vi "svx_Oct_Crop X to scale.vi"(7 "Display State In":T1={"X Scale Width %"=50.0, "Y Scale Height %"=50.0, "X-Axis Range"={"Minimum"=0.0, "Maximum"=10.0}, "Y-Axis Range"={"Minimum"=0.0, "Maximum"=10.0}, "Z-Axis Range"={"Minimum"=0.0, "Maximum"=10.0}, "Plot Color"=0, "Frame Color"=61212, "Background Color"=16252785, "Initial AutoScale Y"=TRUE, "AutoScale X"=2, "AutoScale Y"=2, "AutoScale Z"=2, "Plot Transparency"=FALSE, "X-Axis Name"="Frequency", "Y-Axis Name"="Amplitude", "Z-Axis Name"="", "X-Axis Scaling Factor"={"Offset"=0.0, "Multiplier"=1.0}, "Y-Axis Scaling Factor"={"Offset"=0.0, "Multiplier"=1.0}, "Z-Axis Scaling Factor"={"Offset"=0.0, "Multiplier"=1.0}, "X-Scale Visible"=TRUE, "Y-Scale Visible"=TRUE, "Z-Scale Visible"=TRUE, "X-Scale Label Visible"=TRUE, "Y-Scale Label Visible"=TRUE, "Z-Scale Label Visible"=TRUE, "X-Axis Range Scaled"={"Minimum"=0.0, "Maximum"=10.0}, "Y-Axis Range Scaled"={"Minimum"=0.0, "Maximum"=10.0}, "Z-Axis Range Scaled"={"Minimum"=0.0, "Maximum"=10.0}, "Rev Z Order"=FALSE, "X-Scale Format Str"="%#.4g", "Y-Scale Format Str"="%#.4g", "Z-Scale Format Str"="%#.4g", "Decor color"=12369084, "Scale Range Change"=refnum, "out of state queue"=refnum, "property nodes"=refnum} caption="State", 9 "Cropped Info":cluster{"First Index":i32, "Length":i32}, 11 "Waveform Array In":T2={"z0"=0.0, "dz"=1.0, "Plots"=[]} {"Plots"."Y" format="%.2f"; "Plots"."X" format="%.2f"}) -> (1 "Cropped Info out":cluster{"First Index":i32, "Length":i32}, 3 "Waveform Array Out":T2={"z0"=0.0, "dz"=1.0, "Plots"=[]} {"Plots"."Y" format="%.2f"; "Plots"."X" format="%.2f"})   [LabVIEW 2017, in "SVX Octave Waterfall Graph.xctl"]
uses:
  <vilib>/addons/_XControls/Octave Waterfall Graph/SVX Octave Waterfall Graph.xctl
  <vilib>/addons/_XControls/Octave Waterfall Graph/subVIs/svx_Oct_Waterfall Data.ctl
  <vilib>/addons/_XControls/Octave Waterfall Graph/subVIs/svx_Oct_Waterfall State.ctl
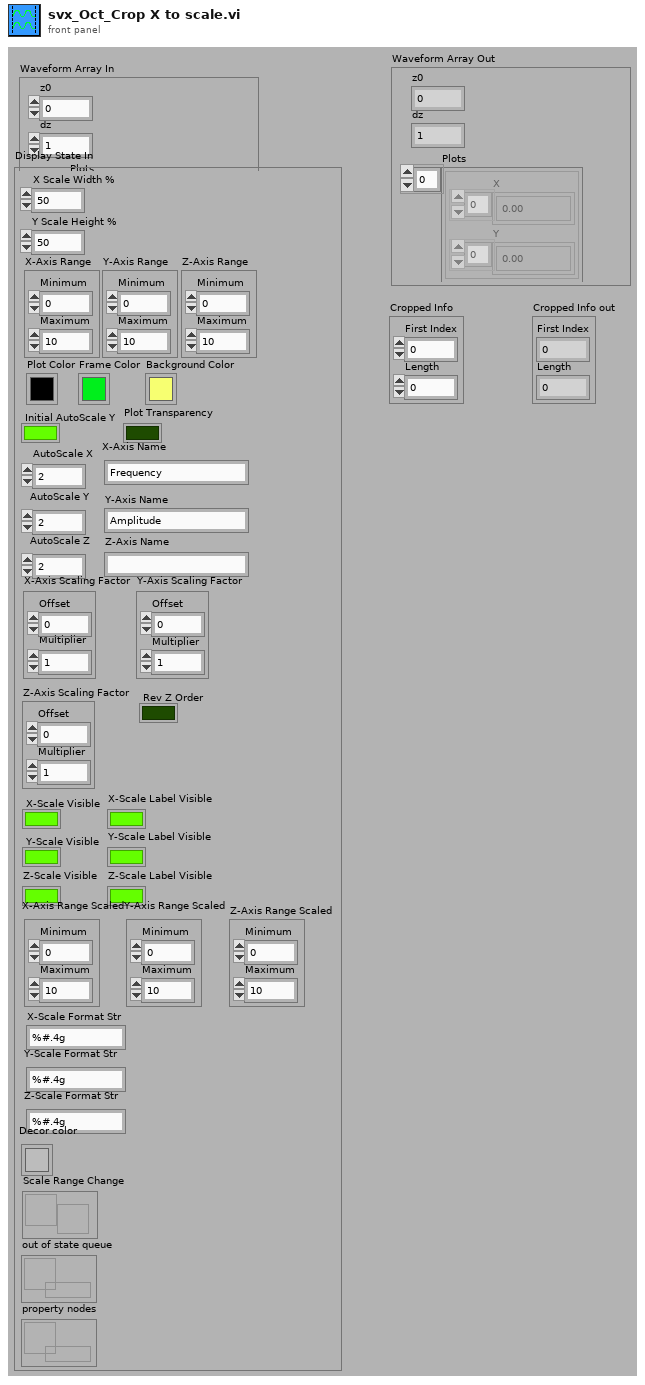
[diagram p1: front panel]
types:
  T1 = typedef "SVX Octave Waterfall Graph.xctl/svx_Oct_Waterfall State.ctl" = cluster{"X Scale Width %":dbl, "Y Scale Height %":dbl, "X-Axis Range":cluster{"Minimum":dbl, "Maximum":dbl}, "Y-Axis Range":cluster{"Minimum":dbl, "Maximum":dbl}, "Z-Axis Range":cluster{"Minimum":dbl, "Maximum":dbl}, "Plot Color":u32, "Frame Color":u32, "Background Color":u32, "Initial AutoScale Y":bool, "AutoScale X":u8, "AutoScale Y":u8, "AutoScale Z":u8, "Plot Transparency":bool, "X-Axis Name":string, "Y-Axis Name":string, "Z-Axis Name":string, "X-Axis Scaling Factor":cluster{"Offset":dbl, "Multiplier":dbl}, "Y-Axis Scaling Factor":cluster{"Offset":dbl, "Multiplier":dbl}, "Z-Axis Scaling Factor":cluster{"Offset":dbl, "Multiplier":dbl}, "X-Scale Visible":bool, "Y-Scale Visible":bool, "Z-Scale Visible":bool, "X-Scale Label Visible":bool, "Y-Scale Label Visible":bool, "Z-Scale Label Visible":bool, "X-Axis Range Scaled":cluster{"Minimum":dbl, "Maximum":dbl}, "Y-Axis Range Scaled":cluster{"Minimum":dbl, "Maximum":dbl}, "Z-Axis Range Scaled":cluster{"Minimum":dbl, "Maximum":dbl}, "Rev Z Order":bool, "X-Scale Format Str":string, "Y-Scale Format Str":string, "Z-Scale Format Str":string, "Decor color":u32, "Scale Range Change":refnum<user-event>, "out of state queue":refnum<queue>, "property nodes":refnum<queue>}
  T2 = typedef "SVX Octave Waterfall Graph.xctl/svx_Oct_Waterfall Data.ctl" = cluster{"z0":dbl, "dz":dbl, "Plots":cluster{"X":dbl[], "Y":dbl[]}[]}
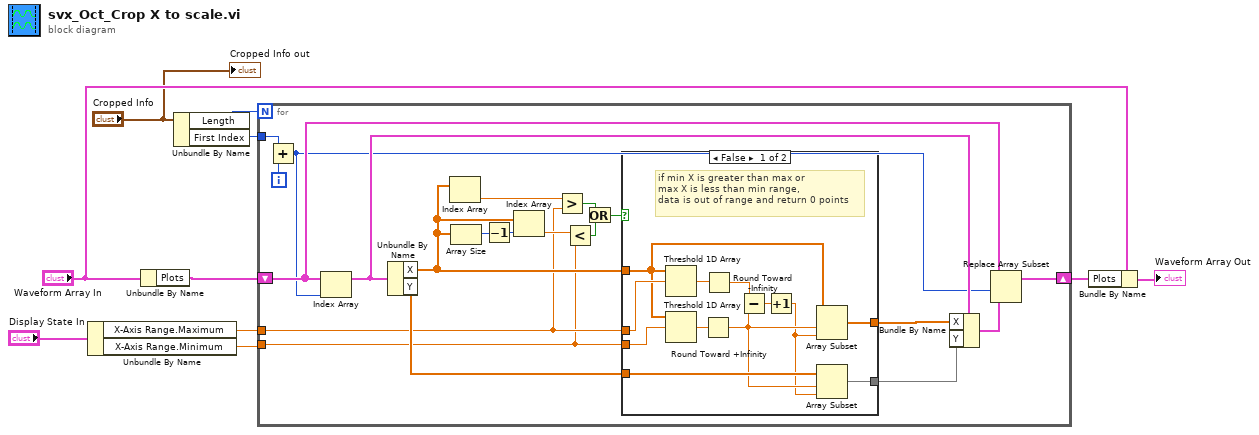
[diagram p0: block diagram]
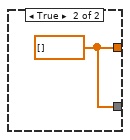
[diagram p2: hidden frame]
diagram:
  n1 = Unbundle By Name("Display State In") -> ("X-Axis Range.Maximum"=w10:dbl, "X-Axis Range.Minimum"=w9:dbl)
  n2 = Unbundle By Name("Waveform Array In") -> ("Plots"=w4:cluster{"X":dbl[], "Y":dbl[]}[])
  n3 = Unbundle By Name("Cropped Info") -> ("Length"=w5:i32, "First Index"=w3:i32)
  n4 = for {
    N: w5 -> [_]
    tunnel: w10 -> [w19]
    tunnel: w9 -> [w18]
    shift-right: [w11] -> w2
    shift-left: w4 -> [w16]
    tunnel: w3 -> [w14]
    i -> [w13]
    n5 = Add(x=w14, y=w13) -> (x+y=w12:i32)
    n6 = Index Array(array=w16, index=w12) -> (element=w17:cluster{"X":dbl[], "Y":dbl[]})
    n7 = Unbundle By Name(w17) -> ("X"=w22:dbl[], "Y"=w29:dbl[])
    n8 = Index Array(array=w22) -> (element=w24:dbl)  [unwired: 1 in]
    n9 = Array Size(array=w22) -> (size(s)=w25:i32)
    n10 = Decrement(x=w25) -> (x-1=w23:i32)
    n11 = Index Array(array=w22, index=w23) -> (element=w21:dbl)
    n12 = Greater?(x=w24, y=w19) -> (0:w26:bool)
    n13 = Less?(x=w21, y=w18) -> (x < y?=w27:bool)
    n14 = Or(x=w26, y=w27) -> (x .or. y?=w20:bool)
    n15 = case shown="False" w20 {
      tunnel: [w39 w43] -> w30
      tunnel: w29 -> [w38 _]
      tunnel: [w36 w43] -> w28
      tunnel: w19 -> [w33 _]
      tunnel: w22 -> [w32 _]
      tunnel: w18 -> [w31 _]
      frame False {
        # "if min X is greater than max or\nmax X is less than min range,\ndata is out of range and return 0 points"
        n16 = Threshold 1D Array(2:w33, 3:w32) -> (0:w41:dbl)  [unwired: 1 in]
        n17 = Threshold 1D Array(2:w31, 3:w32) -> (0:w42:dbl)  [unwired: 1 in]
        n18 = Round Toward +Infinity(x=w42) -> (ceil(x): smallest int >= x=w37:dbl)
        n19 = Round Toward -Infinity(1:w41) -> (0:w40:dbl)
        n20 = Subtract(x=w40, y=w37) -> (x-y=w35:dbl)
        n21 = Increment(x=w35) -> (x+1=w34:dbl)
        n22 = Array Subset(array=w32, index=w37, length=w34) -> (w39:dbl[])
        n23 = Array Subset(array=w38, index=w37, length=w34) -> (w36:dbl[])
      }
      frame True {
        w43 = dbl[] []
      }
    }
    n24 = Bundle By Name(cluster=w17, "X"=w30, "Y"=w28) -> (w15:cluster{"X":dbl[], "Y":dbl[]})
    n25 = Replace Array Subset(array=w16, new element=w15, index=w12) -> (w11:cluster{"X":dbl[], "Y":dbl[]}[])
  }
  n26 = Bundle By Name(cluster="Waveform Array In", "Plots"=w2) -> (→"Waveform Array Out":T2)
  "Cropped Info out" <- "Cropped Info"
